vi "MCores_U16_Noise_Img_Gen-2.vi"(8 "error IN":errorcluster, 9 "[IN] Width":i32, 10 "[IN] Height":i32) -> (0 "error OUT":errorcluster, 2 "[OUT] U16 Pixel Img":u16[][](array[numeric]))   [LabVIEW 2020]
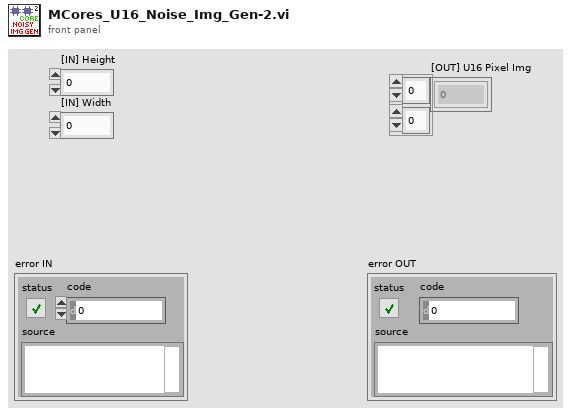
[diagram p1: front panel]
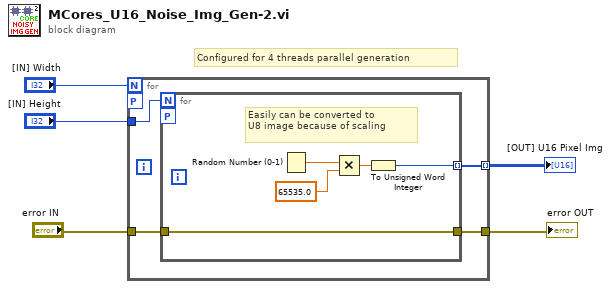
[diagram p0: block diagram]
diagram:
  # "Configured for 4 threads parallel generation"
  n1 = for {
    N: "[IN] Width" -> [_]
    tunnel: "error IN" -> [w9]
    tunnel: [w8] -> w2
    tunnel: "[IN] Height" -> [w7]
    workers-P: _ -> [_]
    tunnel: [w6] -> w1 mode=indexing
    n2 = for {
      N: w7 -> [_]
      tunnel: w9 -> [w14]
      tunnel: [w14] -> w8
      workers-P: _ -> [_]
      tunnel: [w10] -> w6 mode=indexing
      # "Easily can be converted to\nU8 image because of scaling"
      n3 = Random Number (0-1)() -> (number: 0 to 1=w12:dbl)
      n4 = Multiply(x=w12, y=65535.0) -> (x*y=w13:dbl)
      n5 = To Unsigned Word Integer(number=w13) -> (unsigned 16bit integer=w10:u16)
    }
  }
  "error OUT" <- w2
  "[OUT] U16 Pixel Img" <- w1
